vi "Retro Normalized Range Compare 2015.vi"(3 "Y Averages":dbl[](graph), 5 "X Averages":dbl[](graph)) -> (0 "Y Score":dbl, 1 "Ell":bool, 2 "X Score":dbl)   [LabVIEW 2025]
doc: "The input data represents the average pixels set for each row and each column of the possible target. Since targets are expected to have hollow portions, covered in tape, compare the pixels average to the expected min and max values across the target. Higher scores indicate the averages fit the expected profiles."
panel:
  out "Y Results":dbl[][](graph)
  in  "Y Min":dbl[](array[numeric])=[0.1, 0.1, 0.1, 0.1, 0.1, 0.1, 0.1, 0.1, 0.1, 0.1, 0.2, 0.8, 0.5]
  in  "Y Max":dbl[](array[numeric])=[0.4, 0.4, 0.4, 0.4, 0.4, 0.4, 0.4, 0.4, 0.4, 1.0, 1.0, 1.0, 1.0]
  in  "X Min":dbl[](array[numeric])=[0.0, 0.0, 0.0, 0.0, 0.0, 0.0, 0.0, 0.0, 0.0, 0.0, 0.0, 0.0, 0.0, 0.0, 0.0, 0.0, 0.0, 0.0, 0.0, 0.0, 0.0, 0.0, 0.0, 0.0]
  out "X Results":dbl[][](graph)
  in  "X Max":dbl[](array[numeric])=[0.4, 0.4, 0.4, 0.4, 0.4, 0.4, 0.4, 0.4, 0.4, 0.4, 0.4, 0.4, 0.4, 0.4, 0.4, 1.0, 1.0, 1.0, 1.0, 1.0, 1.0, 1.0, 1.0, 1.0]
  # "Measure the average pixel row/column values against the limits, counting how many are between the min and max. \nThe top graphs are pixel columns with the vertical scale flipped to better show what this is measuring.\nThe bottom graphs are still sideways and are the sum of both _| |_ shapes."
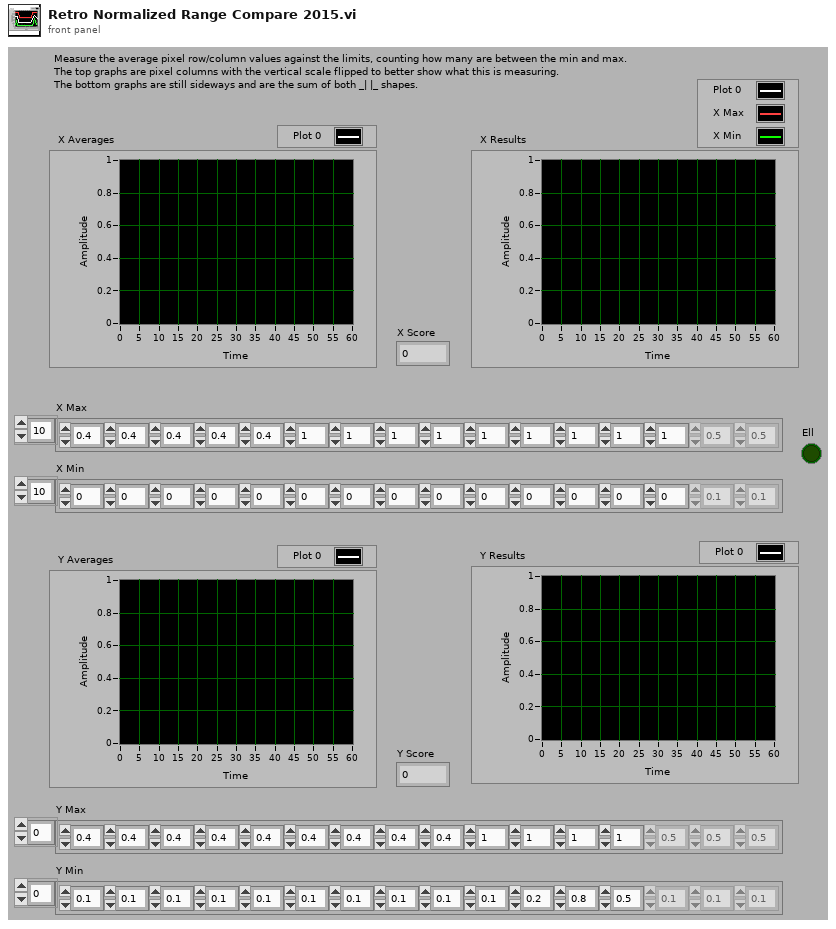
[diagram p1: front panel]
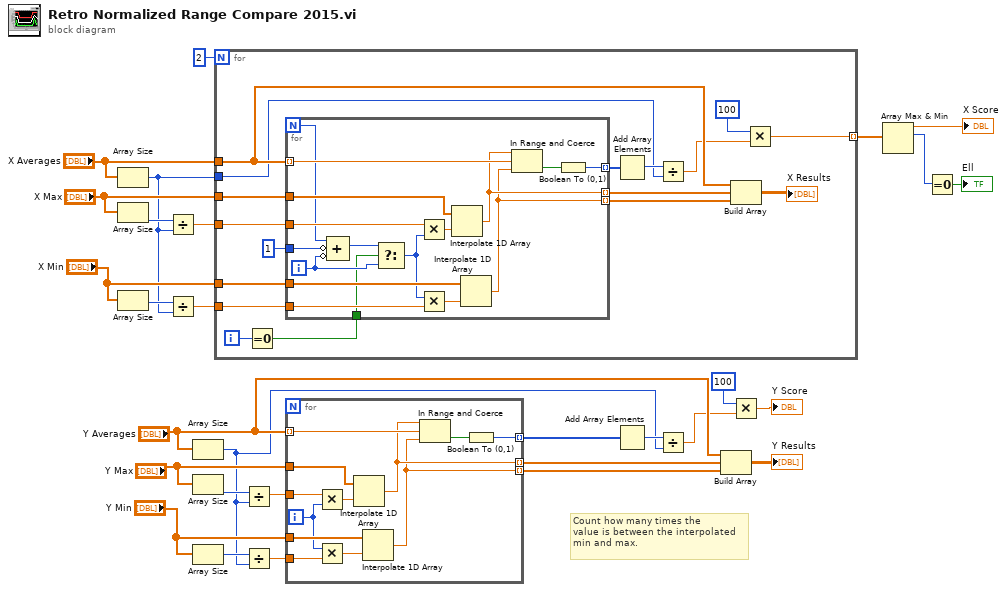
[diagram p0: block diagram]
diagram:
  # "Count how many times the\nvalue is between the interpolated\nmin and max."
  n1 = Array Size(array="X Averages") -> (size(s)=w10:i32)
  n2 = Array Size(array="X Max") -> (size(s)=w27:i32)
  n3 = Array Size(array="X Min") -> (size(s)=w16:i32)
  n4 = Divide(x=w27, y=w10) -> (x/y=w26:dbl)
  n5 = Divide(x=w16, y=w10) -> (x/y=w14:dbl)
  n6 = Array Size(array="Y Averages") -> (size(s)=w9:i32)
  n7 = Array Size(array="Y Max") -> (size(s)=w25:i32)
  n8 = Array Size(array="Y Min") -> (size(s)=w18:i32)
  n9 = for {
    N: 2 -> [_]
    tunnel: "X Averages" -> [w43]
    tunnel: "X Max" -> [w42]
    tunnel: w26 -> [w41]
    tunnel: "X Min" -> [w40]
    tunnel: w14 -> [w39]
    tunnel: w10 -> [w36]
    tunnel: [w30] -> w5 mode=indexing
    i -> [w32]
    n10 = Equal To 0?(x=w32) -> (x = 0?=w31:bool)
    n11 = for {
      N -> [w52]
      tunnel: w43 -> [w63] mode=indexing
      tunnel: w42 -> [w61]
      tunnel: [w60] -> w46 mode=indexing
      tunnel: [w57] -> w45 mode=indexing
      tunnel: w41 -> [w62]
      tunnel: w40 -> [w59]
      tunnel: w39 -> [w56]
      tunnel: [w53] -> w38 mode=indexing
      tunnel: 1 -> [w49]
      tunnel: w31 -> [w47]
      i -> [w48]
      n12 = Compound Arithmetic op=ADD(w52, invert w49, invert w48) -> (w50:i32)
      n13 = Select(t=w50, s=w47, f=w48) -> (s? t:f=w51:i32)
      n14 = Multiply(x=w62, y=w51) -> (x*y=w58:dbl)
      n15 = Multiply(x=w51, y=w56) -> (x*y=w55:dbl)
      n16 = Interpolate 1D Array(1:w58, 2:w61) -> (0:w60:dbl)
      n17 = Interpolate 1D Array(1:w55, 2:w59) -> (0:w57:dbl)
      n18 = In Range and Coerce(upper limit=w60, x=w63, lower limit=w57) -> (In Range?=w54:bool)  [unwired: 1 out]
      n19 = Boolean To (0,1)(Boolean=w54) -> (0, 1=w53:i16)
    }
    n20 = Add Array Elements(numeric array=w38) -> (sum=w37:i16)
    n21 = Divide(x=w37, y=w36) -> (x/y=w35:dbl)
    n22 = Build Array(w43, w46, w45) -> (→"X Results":dbl[][])
    n23 = Multiply(x=100, y=w35) -> (x*y=w30:dbl)
  }
  n24 = Divide(x=w25, y=w9) -> (x/y=w23:dbl)
  n25 = Divide(x=w18, y=w9) -> (x/y=w13:dbl)
  n26 = for {
    tunnel: "Y Averages" -> [w75] mode=indexing
    tunnel: "Y Max" -> [w73]
    tunnel: [w72] -> w21 mode=indexing
    tunnel: [w69] -> w20 mode=indexing
    tunnel: w23 -> [w74]
    tunnel: "Y Min" -> [w71]
    tunnel: w13 -> [w66]
    tunnel: [w64] -> w12 mode=indexing
    i -> [w68]
    n27 = Multiply(x=w74, y=w68) -> (x*y=w70:dbl)
    n28 = Multiply(x=w68, y=w66) -> (x*y=w67:dbl)
    n29 = Interpolate 1D Array(1:w70, 2:w73) -> (0:w72:dbl)
    n30 = Interpolate 1D Array(1:w67, 2:w71) -> (0:w69:dbl)
    n31 = In Range and Coerce(upper limit=w72, x=w75, lower limit=w69) -> (In Range?=w65:bool)  [unwired: 1 out]
    n32 = Boolean To (0,1)(Boolean=w65) -> (0, 1=w64:i16)
  }
  n33 = Add Array Elements(numeric array=w12) -> (sum=w11:i16)
  n34 = Divide(x=w11, y=w9) -> (x/y=w8:dbl)
  n35 = Build Array("Y Averages", w21, w20) -> (→"Y Results":dbl[][])
  n36 = Multiply(x=100, y=w8) -> (x*y=→"Y Score":dbl)
  n37 = Array Max & Min(array=w5) -> (max value=→"X Score":dbl, max index (indices)=w3:i32)  [unwired: 2 out]
  n38 = Equal To 0?(x=w3) -> (x = 0?=→"Ell":bool)
